vi "onTestExecution.vi"(6 "timeout (2000 ms)":i32=2000, 7 "Name":string, 8 "error in (no error)":errorcluster, 11 "Test Runner.BrokenTests in":refnum<class "Test Runner.BrokenTest.lvclass">) -> (0 "error out":errorcluster, 3 "Test Runner.BrokenTests":refnum<class "Test Runner.BrokenTest.lvclass">)   [LabVIEW 2013, in "Test Runner.BrokenTest.lvclass"]
uses:
  Test Runner.BrokenTest.lvclass
  classes/Test Runner/Test Runner.lvclass/Test Runner.ctl
  classes/Assert/Assert Error.vi
  classes/Assert/Assert Not Error.vi
  classes/Test/Test.lvclass
  classes/Assert/Assert.lvclass
  classes/Test Runner/Test Runner.lvclass
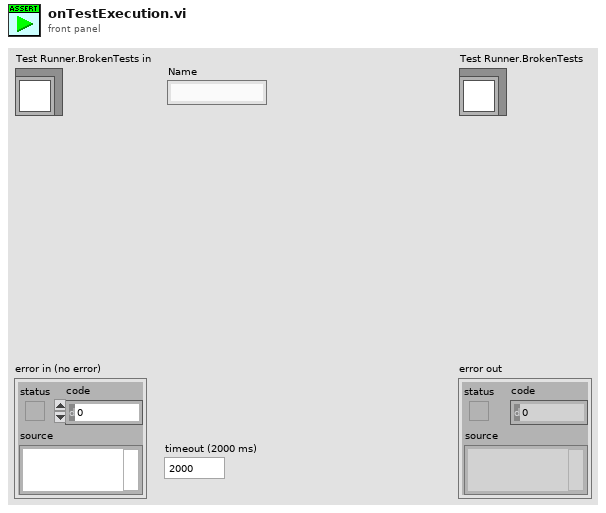
[diagram p1: front panel]
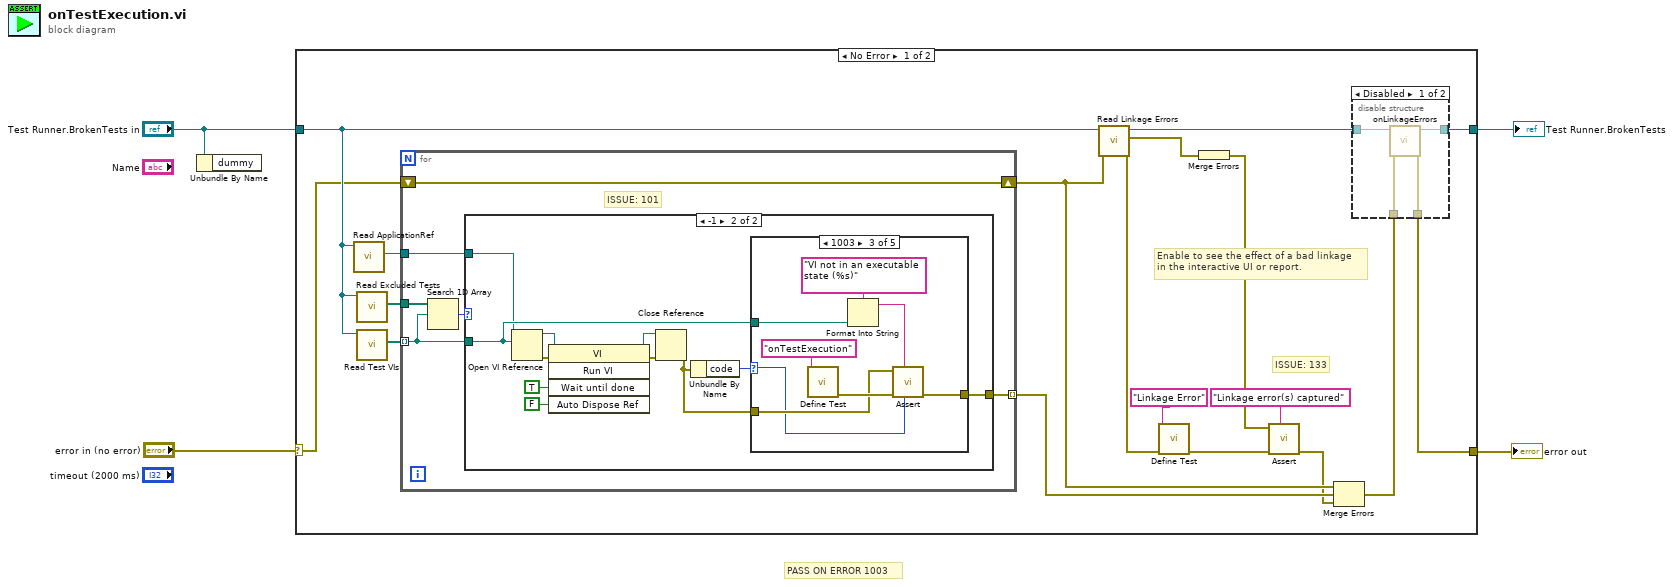
[diagram p0: block diagram]
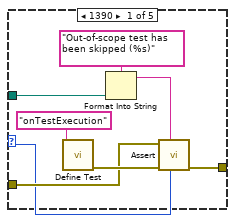
[diagram p4: hidden frame]
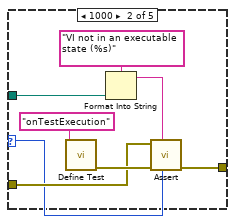
[diagram p5: hidden frame]
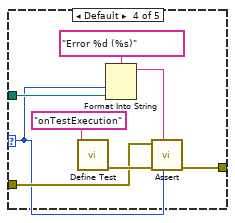
[diagram p6: hidden frame]
diagram:
  # "PASS ON ERROR 1003"
  n1 = Unbundle By Name("Test Runner.BrokenTests in") -> ()  [unwired: 1 out]
  n2 = case shown="No Error" "error in (no error)" {
    selector: "error in (no error)" -> [w11 w79]
    tunnel: "Test Runner.BrokenTests in" -> [w12 w80]
    tunnel: [w7 w80] -> w3
    tunnel: [w6 w79] -> w1
    frame No Error {
      # "ISSUE: 133"
      # "Enable to see the effect of a bad linkage\nin the interactive UI or report."
      n3 = call "Read ApplicationRef.vi"("Test Runner in"=w12) -> ("Application"=w13:refnum<vi>)  [unwired: 8 in, 2 out]
      n4 = call "Read Excluded Tests.vi"("Test Runner in"=w12) -> ("Excluded Tests"=w15:path[])  [unwired: 8 in, 2 out]
      n5 = call "Read Test VIs.vi"("Test Runner in"=w12) -> ("Test VIs"=w14:path[])  [unwired: 8 in, 2 out]
      n6 = for {
        tunnel: w14 -> [w33] mode=indexing
        tunnel: [w32] -> w16 mode=indexing
        tunnel: w15 -> [w34]
        tunnel: w13 -> [w30]
        shift-right: [w29] -> w10
        shift-left: w11 -> [w29]
        # "ISSUE: 101"
        n7 = Search 1D Array(1D array=w34, element=w33) -> (index of element=w31:i32)  [unwired: 1 in]
        n8 = case shown="-1" w31 {
          tunnel: w33 -> [_ w37]
          tunnel: [_ w36] -> w32
          tunnel: w30 -> [_ w35]
          frame Default {
            # "Test is part of the exclusion list"
          }
          frame -1 {
            n9 = Open VI Reference(application reference (local)=w35, vi path=w37) -> (vi reference=w38:refnum<vi>, error out=w45:errorcluster)  [unwired: 4 in]
            n10 = invoke on="Invoke Node" class="VI" method="Run VI"(reference=w38, error in=w45, "Wait until done"=TRUE ("Wait Until Done"), "Auto Dispose Ref"=FALSE ("Auto Dispose Reference")) -> (reference out=w41:refnum<vi>, error out=w40:errorcluster)  [unwired: 1 in, 3 out]
            n11 = Close Reference(reference=w41, error in (no error)=w40) -> (error out=w39:errorcluster)
            n12 = Unbundle By Name(w39) -> ("code"=w42:i32)
            n13 = case shown="1003" w42 {
              selector: w42 -> [w46 w54 w62 w70 _]
              tunnel: w39 -> [w47 w55 w63 w71 w78]
              tunnel: [w49 w57 w65 w74 w78] -> w36
              tunnel: w37 -> [w53 w61 w69 w77 _]
              frame 1390 {
                n14 = call "Define Test.vi"("Label (VI Title)"="onTestExecution" ("Label")) -> ("error out"=w50:errorcluster)  [unwired: 10 in]
                n15 = Format Into String(format string="Out-of-scope test has been skipped (%s)" ("Label"), w53) -> (resulting string=w48:string)  [unwired: 2 in, 1 out]
                n16 = call-poly "Assert.vi"("error code (1)"=w46, "Label"=w48, "error in (no error)"=w50, "Not Error?"=w47) -> ("error out"=w49:errorcluster)  [unwired: 7 in]
              }
              frame 1000 {
                n17 = call "Define Test.vi"("Label (VI Title)"="onTestExecution" ("Label")) -> ("error out"=w58:errorcluster)  [unwired: 10 in]
                n18 = Format Into String(format string="VI not in an executable state (%s)" ("Label"), w61) -> (resulting string=w56:string)  [unwired: 2 in, 1 out]
                n19 = call-poly "Assert.vi"("error code (1)"=w54, "Label"=w56, "error in (no error)"=w58, "Not Error?"=w55) -> ("error out"=w57:errorcluster)  [unwired: 7 in]
              }
              frame 1003 {
                n20 = call "Define Test.vi"("Label (VI Title)"="onTestExecution" ("Label")) -> ("error out"=w66:errorcluster)  [unwired: 10 in]
                n21 = Format Into String(format string="VI not in an executable state (%s)" ("Label"), w69) -> (resulting string=w64:string)  [unwired: 2 in, 1 out]
                n22 = call-poly "Assert.vi"("error code (1)"=w62, "Label"=w64, "error in (no error)"=w66, "Error?"=w63) -> ("error out"=w65:errorcluster)  [unwired: 7 in]
              }
              frame Default {
                n23 = call "Define Test.vi"("Label (VI Title)"="onTestExecution" ("Label")) -> ("error out"=w72:errorcluster)  [unwired: 10 in]
                n24 = Format Into String(format string="Error %d (%s)" ("Label"), w70, w77) -> (resulting string=w73:string)  [unwired: 2 in, 1 out]
                n25 = call-poly "Assert.vi"("error code (1)"=w70, "Label"=w73, "error in (no error)"=w72, "Not Error?"=w71) -> ("error out"=w74:errorcluster)  [unwired: 7 in]
              }
              frame 0 {
              }
            }
          }
        }
      }
      n26 = call "Read Linkage Errors.vi"("error in (no error)"=w10, "Test Runner in"=w12) -> ("error out"=w17:errorcluster, "Linkage Errors"=w19:errorcluster[], "Test Runner out"=w8:refnum<class "Test Runner.BrokenTest.lvclass">)  [unwired: 7 in]
      n27 = call "Define Test.vi"("error in (no error)"=w17, "Label (VI Title)"="Linkage Error" ("Label")) -> ("error out"=w21:errorcluster)  [unwired: 9 in]
      n28 = Merge Errors(w19) -> (w18:errorcluster)
      n29 = call-poly "Assert.vi"("Label"="Linkage error(s) captured", "error in (no error)"=w21, "Error?"=w18) -> ("error out"=w9:errorcluster)  [unwired: 8 in]
      n30 = Merge Errors(w10, w16, w9) -> (w5:errorcluster)
      n31 = disable-structure shown="Disabled" {
        disable-tunnel: w8 -> [w26 w28]
        disable-tunnel: [w25 w28] -> w7
        disable-tunnel: [w24 w27] -> w6
        disable-tunnel: w5 -> [w23 w27]
        frame Disabled {
          n32 = call-dynamic "onLinkageErrors.vi"("error in (no error)"=w23, "Test Runner in"=w26) -> ("error out"=w24:errorcluster, "Test Runner out"=w25:refnum<class "Test Runner.BrokenTest.lvclass">)  [unwired: 8 in]
        }
        frame Enabled {
        }
      }
    }
    frame Error {
    }
  }
  "error out" <- w1
  "Test Runner.BrokenTests" <- w3
